vi "gui_control.vi"() -> ()   [LabVIEW 2020]
uses:
  <vilib>/Instr/_visa.llb/VISA Configure Serial Port (Instr).vi
panel:
  out "Connected":bool
  out "Response":string
  in  "CONNECTION":bool
  out "Bytes Read":u32
  in  "VISA Resource":refnum<visa-resource-name>="COM1"
  in  "Tab Control":enum32{"Page 1", "Page 2"}(tab)
  in  "End":timestamp caption="Day End" format="%<%H:%M>T"
  in  "Start":timestamp caption="Day Start" format="%<%H:%M>T"
  in  "SEND LED":bool caption="Boolean"
  out "Color Box":u32(colorbox)
  in  "R":u8
  in  "G":u8
  in  "B":u8
  in  "SEND RTC":bool caption="Boolean"
  in  "SEND INT":bool caption="Boolean"
  in  "INT 2":u8 caption="Brightness"
  out "Humidity":string caption="Humidity (%)"
  out "Temp":string caption="Temp (°C)"
  out "Temp 2":string caption="Temp (°C)"
  in  "B 2":u8 caption="B"
  in  "G 2":u8 caption="G"
  in  "R 2":u8 caption="R"
  out "Color Box 2":u32(colorbox)
  in  "SEND RTC 2":bool caption="Boolean"
  in  "SEND LED 2":bool caption="Boolean"
  in  "End 2":timestamp caption="Day End" format="%<%H:%M>T"
  in  "Start 2":timestamp caption="Day Start" format="%<%H:%M>T"
  in  "SEND INT 2":bool caption="Boolean"
  in  "INT":u8 caption="Brightness"
  out "Humidity 2":string caption="Humidity (%)"
  # "Serial Monitor"
  # "--- Box 1 ---"
  # "Auto LED Timer"
  # "Manual Color Control"
  # "Climate Readings"
  # "--- Box 2 ---"
  # "Auto LED Timer"
  # "Manual Color Control"
  # "Climate Readings"
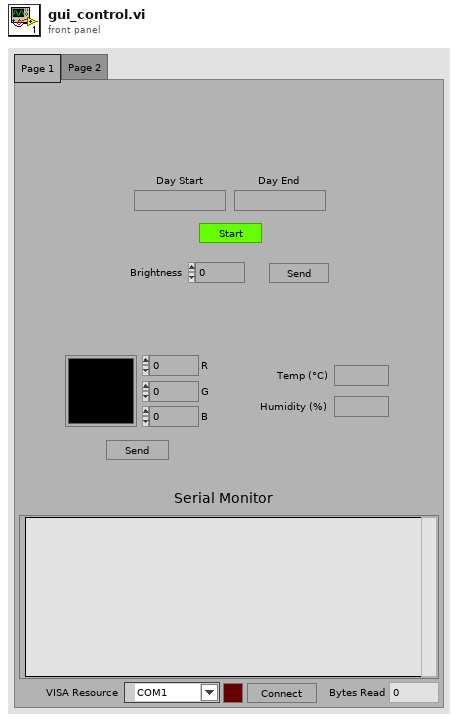
[diagram p1: front panel]
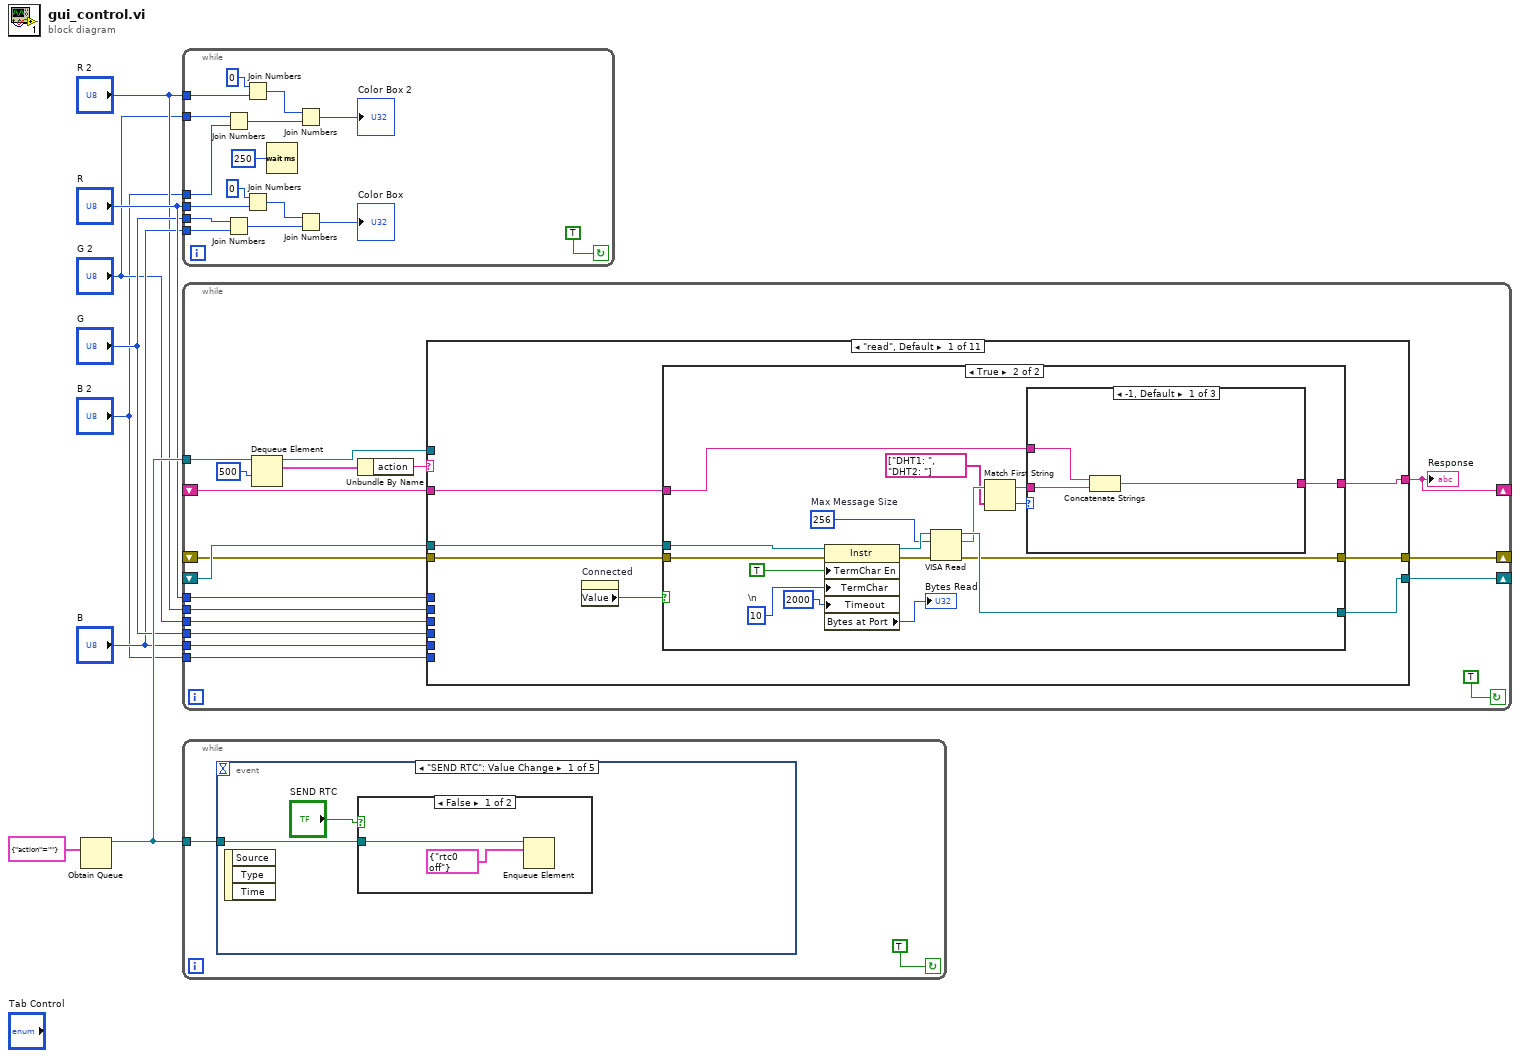
[diagram p0: block diagram]
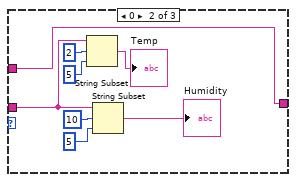
[diagram p3: hidden frame]
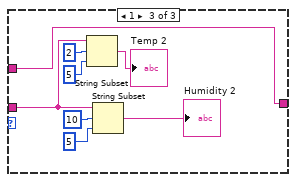
[diagram p4: hidden frame]
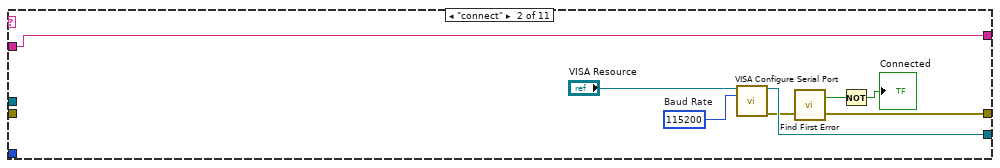
[diagram p5: hidden frame]
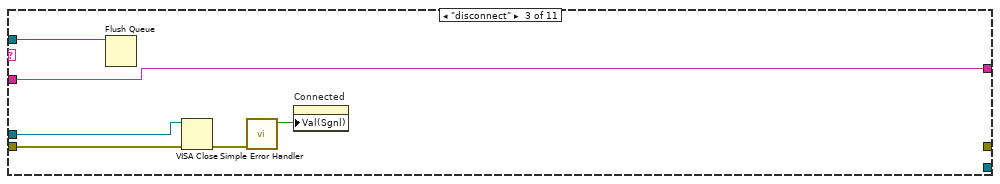
[diagram p6: hidden frame]
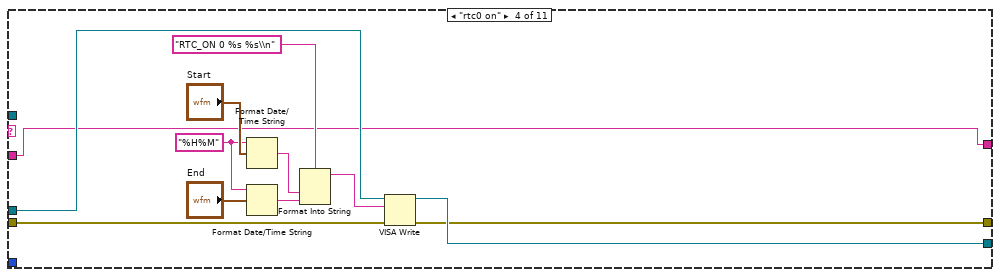
[diagram p7: hidden frame]
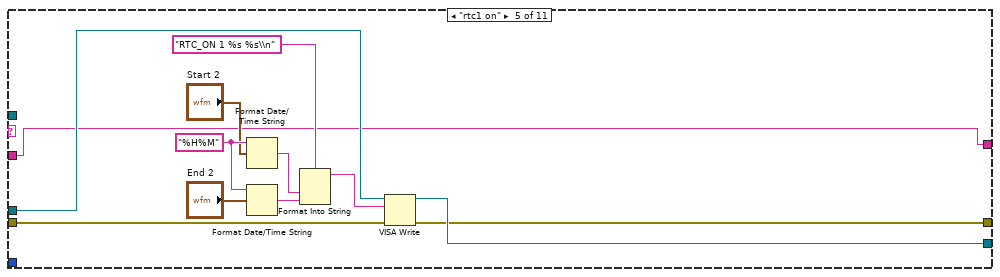
[diagram p8: hidden frame]
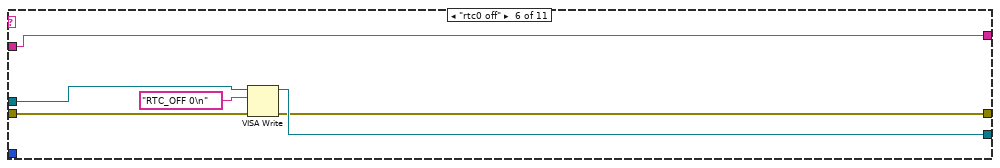
[diagram p9: hidden frame]
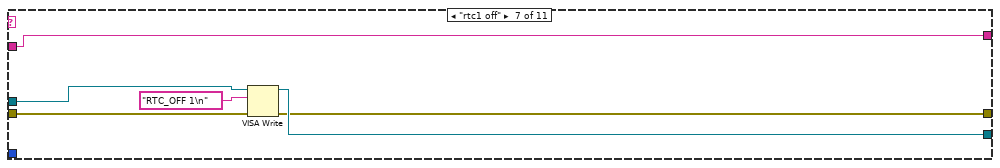
[diagram p10: hidden frame]
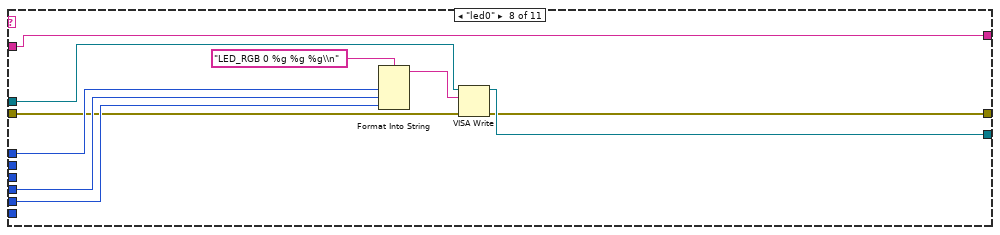
[diagram p11: hidden frame]
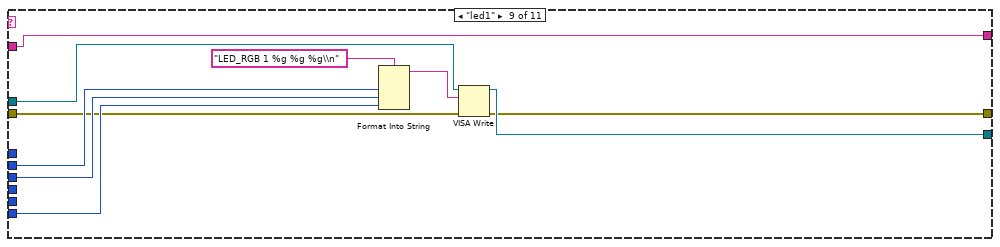
[diagram p12: hidden frame]
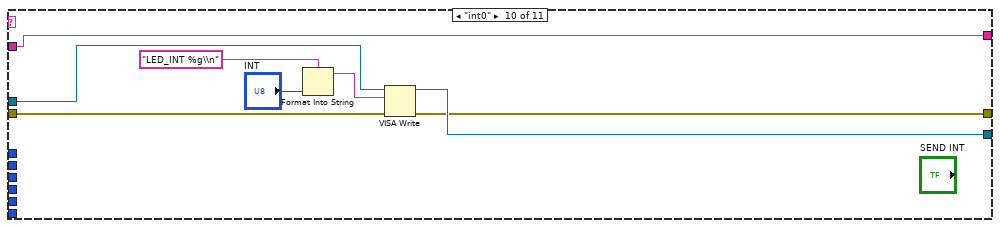
[diagram p13: hidden frame]
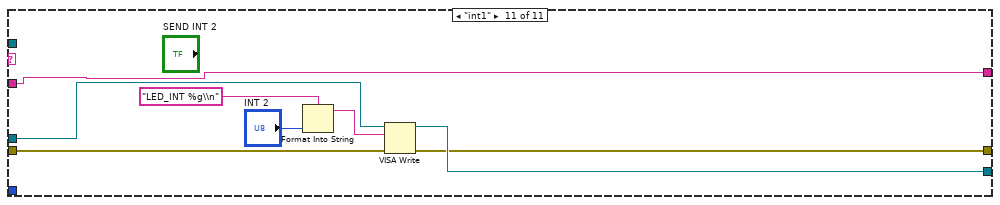
[diagram p14: hidden frame]
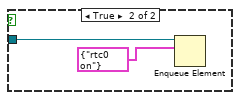
[diagram p15: hidden frame]
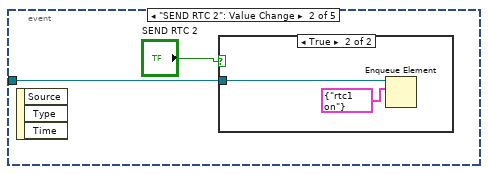
[diagram p16: hidden frame]
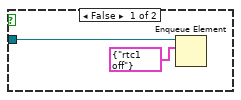
[diagram p17: hidden frame]
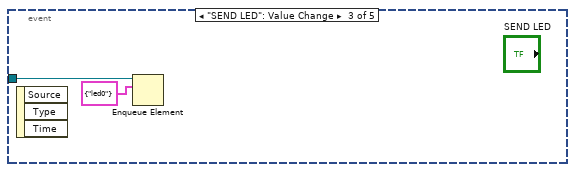
[diagram p18: hidden frame]
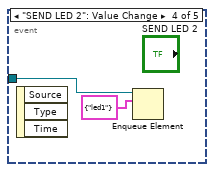
[diagram p19: hidden frame]
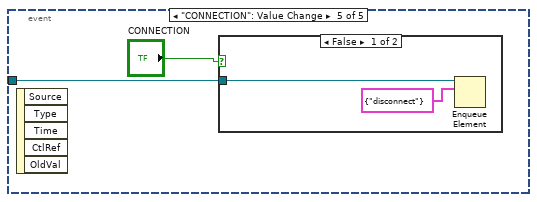
[diagram p20: hidden frame]
diagram:
  n1 = Obtain Queue(element data type=cluster{"action":string} {"action"=""}) -> (queue out=w7:refnum<queue>)  [unwired: 4 in, 2 out]
  n2 = while {
    tunnel: "R" -> [w18]
    tunnel: "G" -> [w17]
    tunnel: "B" -> [w16]
    tunnel: "R 2" -> [w14]
    tunnel: "G 2" -> [w12]
    tunnel: "B 2" -> [w11]
    stop <- TRUE continue-if-true
    n3 = Join Numbers(hi=w12, lo=w11) -> ((hi.lo)=w10:u16)
    n4 = Join Numbers(hi=w17, lo=w16) -> ((hi.lo)=w20:u16)
    n5 = Join Numbers(hi=u8 0, lo=w14) -> ((hi.lo)=w9:u16)
    n6 = Join Numbers(hi=u8 0, lo=w18) -> ((hi.lo)=w21:u16)
    n7 = Wait (ms)(milliseconds to wait=u32 250) -> ()  [unwired: 1 out]
    n8 = Join Numbers(hi=w9, lo=w10) -> ((hi.lo)=→"Color Box 2":u32)
    n9 = Join Numbers(hi=w21, lo=w20) -> ((hi.lo)=→"Color Box":u32)
  }
  n10 = while {
    tunnel: w7 -> [w42]
    shift-right: [w37] -> _
    shift-left: _ -> [w36]
    shift-right: [w35] -> _
    shift-left: _ -> [w34]
    tunnel: "R" -> [w33]
    tunnel: "G" -> [w32]
    tunnel: "B" -> [w31]
    tunnel: "R 2" -> [w30]
    tunnel: "G 2" -> [w29]
    tunnel: "B 2" -> [w28]
    shift-right: [w26] -> _
    shift-left: _ -> [w27]
    stop <- TRUE continue-if-true
    n11 = Dequeue Element(queue=w42, timeout in ms (-1)=500) -> (queue out=w38:refnum<queue>, element=w40:cluster{"action":string})  [unwired: 1 in, 2 out]
    n12 = Unbundle By Name(w40) -> ("action"=w39:string)
    n13 = case shown="\"read\", Default" w39 {
      tunnel: w38 -> [_ _ w97 _ _ _ _ _ _ _ _]
      tunnel: [w43 w92 _ w104 w117 w129 w135 w143 w153 w160 w169] -> w37
      tunnel: w36 -> [w49 _ w100 w105 w116 w130 w136 w144 w154 w161 w170]
      tunnel: [w47 w90 _ w102 w114 w127 w133 w138 w148 w158 w166] -> w35
      tunnel: w34 -> [w48 _ w98 w103 w115 w128 w134 w139 w149 w159 w167]
      tunnel: w33 -> [_ _ _ _ _ _ _ w142 _ _ _]
      tunnel: w32 -> [_ _ _ _ _ _ _ w141 _ _ _]
      tunnel: w31 -> [_ _ _ _ _ _ _ w140 _ _ _]
      tunnel: w30 -> [_ _ _ _ _ _ _ _ w152 _ _]
      tunnel: w29 -> [_ _ _ _ _ _ _ _ w151 _ _]
      tunnel: w28 -> [_ _ _ _ _ _ _ _ w150 _ _]
      tunnel: [w45 w87 w95 w101 w113 w126 w132 w137 w147 w157 w165] -> w26
      tunnel: w27 -> [w46 w87 w95 w101 w113 w126 w132 w137 w147 w157 w165]
      frame "read", Default {
        n14 = property on="Connected" class="Bool (strict)"() -> ("Value"=w44:bool)  [unwired: 2 in, 2 out]
        n15 = case shown="True" w44 {
          tunnel: w49 -> [_ w60]
          tunnel: w48 -> [w50 w59]
          tunnel: [w50 w57] -> w47
          tunnel: w46 -> [_ w52]
          tunnel: [_ w51] -> w45
          tunnel: [_ w58] -> w43
          frame False {
          }
          frame True {
            w64 = u32 256  # Max Message Size
            w62 = u8 10  # \n
            n16 = property class="Instr"(reference=w60, error in=w59, "TermChar En"=TRUE ("Message Based Settings:Termination Character Enable"), "TermChar"=w62, "Timeout"=u32 2000 ("General Settings:Timeout Value")) -> (reference out=w67:refnum<visa-resource-name>, error out=w66:errorcluster, "Bytes at Port"=→"Bytes Read":u32)
            n17 = VISA Read(VISA resource name=w67, byte count=w64, error in (no error)=w66) -> (VISA resource name out=w58:refnum<visa-resource-name>, read buffer=w56:string, error out=w57:errorcluster)  [unwired: 1 out]
            n18 = Match First String(2:string[] ["DHT1: ", "DHT2: "], 3:w56) -> (0:w55:i32, 1:w53:string)
            n19 = case shown="-1, Default" w55 {
              tunnel: w53 -> [w68 w72 w81]
              tunnel: w52 -> [w70 w78 w86]
              tunnel: [w69 w78 w86] -> w51
              frame -1, Default {
                n20 = Concatenate Strings(w70, w68) -> (w69:string)
              }
              frame 0 {
                n21 = String Subset(string=w72, offset (0)=2, length (rest)=5) -> (substring=→"Temp":string)
                n22 = String Subset(string=w72, offset (0)=10, length (rest)=5) -> (substring=→"Humidity":string)
              }
              frame 1 {
                n23 = String Subset(string=w81, offset (0)=2, length (rest)=5) -> (substring=→"Temp 2":string)
                n24 = String Subset(string=w81, offset (0)=10, length (rest)=5) -> (substring=→"Humidity 2":string)
              }
            }
          }
        }
      }
      frame "connect" {
        w93 = u32 115200  # Baud Rate
        n25 = call-poly "VISA Configure Serial Port"("VISA resource name"="VISA Resource", "baud rate (9600)"=w93) -> ("VISA resource name out"=w92:refnum<visa-resource-name>, "error out"=w91:errorcluster)  [unwired: 7 in, 5 out]
        n26 = call <vilib>:"Find First Error.vi"("error in (no error)"=w91) -> ("error out"=w90:errorcluster, "error?"=w89:bool)  [unwired: 3 in]
        n27 = Not(x=w89) -> (.not. x?=→"Connected":bool)
      }
      frame "disconnect" {
        n28 = Flush Queue(queue=w97) -> ()  [unwired: 1 in, 3 out]
        n29 = VISA Close(VISA resource name=w100, error in (no error)=w98) -> (error out=w99:errorcluster)
        n30 = call <vilib>:"Simple Error Handler.vi"("error in (no error)"=w99) -> ("error?"=w96:bool)  [unwired: 1 in, 7 out]
        n31 = property on="Connected" class="Bool (strict)"("Val(Sgnl)"=w96) -> ()  [unwired: 2 in, 2 out]
      }
      frame "rtc0 on" {
        w106 = "%H%M"
        n32 = Format Date/Time String(time format string (%c)=w106, seconds (now)="Start") -> (date/time string=w112:string)  [unwired: 1 in]
        n33 = Format Date/Time String(time format string (%c)=w106, seconds (now)="End") -> (date/time string=w111:string)  [unwired: 1 in]
        n34 = Format Into String(format string="RTC_ON 0 %s %s\\n", w112, w111) -> (resulting string=w108:string)  [unwired: 2 in, 1 out]
        n35 = VISA Write(VISA resource name=w105, write buffer=w108, error in (no error)=w103) -> (VISA resource name out=w104:refnum<visa-resource-name>, error out=w102:errorcluster)  [unwired: 1 out]
      }
      frame "rtc1 on" {
        w122 = "%H%M"
        n36 = Format Date/Time String(time format string (%c)=w122, seconds (now)="Start 2") -> (date/time string=w120:string)  [unwired: 1 in]
        n37 = Format Date/Time String(time format string (%c)=w122, seconds (now)="End 2") -> (date/time string=w121:string)  [unwired: 1 in]
        n38 = Format Into String(format string="RTC_ON 1 %s %s\\n", w120, w121) -> (resulting string=w123:string)  [unwired: 2 in, 1 out]
        n39 = VISA Write(VISA resource name=w116, write buffer=w123, error in (no error)=w115) -> (VISA resource name out=w117:refnum<visa-resource-name>, error out=w114:errorcluster)  [unwired: 1 out]
      }
      frame "rtc0 off" {
        n40 = VISA Write(VISA resource name=w130, write buffer="RTC_OFF 0\n" ("format string"), error in (no error)=w128) -> (VISA resource name out=w129:refnum<visa-resource-name>, error out=w127:errorcluster)  [unwired: 1 out]
      }
      frame "rtc1 off" {
        n41 = VISA Write(VISA resource name=w136, write buffer="RTC_OFF 1\n" ("format string"), error in (no error)=w134) -> (VISA resource name out=w135:refnum<visa-resource-name>, error out=w133:errorcluster)  [unwired: 1 out]
      }
      frame "led0" {
        n42 = Format Into String(format string="LED_RGB 0 %g %g %g\\n", w142, w141, w140) -> (resulting string=w145:string)  [unwired: 2 in, 1 out]
        n43 = VISA Write(VISA resource name=w144, write buffer=w145, error in (no error)=w139) -> (VISA resource name out=w143:refnum<visa-resource-name>, error out=w138:errorcluster)  [unwired: 1 out]
      }
      frame "led1" {
        n44 = Format Into String(format string="LED_RGB 1 %g %g %g\\n", w152, w151, w150) -> (resulting string=w155:string)  [unwired: 2 in, 1 out]
        n45 = VISA Write(VISA resource name=w154, write buffer=w155, error in (no error)=w149) -> (VISA resource name out=w153:refnum<visa-resource-name>, error out=w148:errorcluster)  [unwired: 1 out]
      }
      frame "int0" {
        n46 = Format Into String(format string="LED_INT %g\\n", "INT") -> (resulting string=w162:string)  [unwired: 2 in, 1 out]
        n47 = VISA Write(VISA resource name=w161, write buffer=w162, error in (no error)=w159) -> (VISA resource name out=w160:refnum<visa-resource-name>, error out=w158:errorcluster)  [unwired: 1 out]
      }
      frame "int1" {
        n48 = Format Into String(format string="LED_INT %g\\n", "INT 2") -> (resulting string=w171:string)  [unwired: 2 in, 1 out]
        n49 = VISA Write(VISA resource name=w170, write buffer=w171, error in (no error)=w167) -> (VISA resource name out=w169:refnum<visa-resource-name>, error out=w166:errorcluster)  [unwired: 1 out]
      }
    }
    "Response" <- w26
  }
  n50 = while {
    tunnel: w7 -> [w174]
    stop <- TRUE continue-if-true
    n51 = event shown="[0] \"SEND RTC\": Value Change" {
      selector: _ -> [_ _ _ _ _]
      dyn-events: _ -> [_ _ _ _ _]
      timeout: _ -> [_ _ _ _ _]
      tunnel: w174 -> [w175 w181 w187 w189 w192]
      event "SEND RTC": Value Change {
        n52 = event-data() -> ()  [unwired: 1 in, 3 out]
        n53 = case shown="False" "SEND RTC" {
          tunnel: w175 -> [w177 w179]
          frame False {
            n54 = Enqueue Element(queue=w177, element=cluster{"action":string} {"action"="rtc0 off"}) -> ()  [unwired: 2 in, 3 out]
          }
          frame True {
            n55 = Enqueue Element(queue=w179, element=cluster{"action":string} {"action"="rtc0 on"}) -> ()  [unwired: 2 in, 3 out]
          }
        }
      }
      event "SEND RTC 2": Value Change {
        n56 = event-data() -> ()  [unwired: 1 in, 3 out]
        n57 = case shown="True" "SEND RTC 2" {
          tunnel: w181 -> [w183 w185]
          frame False {
            n58 = Enqueue Element(queue=w183, element=cluster{"action":string} {"action"="rtc1 off"}) -> ()  [unwired: 2 in, 3 out]
          }
          frame True {
            n59 = Enqueue Element(queue=w185, element=cluster{"action":string} {"action"="rtc1 on"}) -> ()  [unwired: 2 in, 3 out]
          }
        }
      }
      event "SEND LED": Value Change {
        n60 = event-data() -> ()  [unwired: 1 in, 3 out]
        n61 = Enqueue Element(queue=w187, element=cluster{"action":string} {"action"="led0"}) -> ()  [unwired: 2 in, 3 out]
      }
      event "SEND LED 2": Value Change {
        n62 = event-data() -> ()  [unwired: 1 in, 3 out]
        n63 = Enqueue Element(queue=w189, element=cluster{"action":string} {"action"="led1"}) -> ()  [unwired: 2 in, 3 out]
      }
      event "CONNECTION": Value Change {
        n64 = event-data() -> ()  [unwired: 1 in, 5 out]
        n65 = case shown="False" "CONNECTION" {
          tunnel: w192 -> [w193 w196]
          frame False {
            n66 = Enqueue Element(queue=w193, element=cluster{"action":string} {"action"="disconnect"}) -> ()  [unwired: 2 in, 3 out]
          }
          frame True {
            n67 = Enqueue Element(queue=w196, element=cluster{"action":string} {"action"="connect"}) -> ()  [unwired: 2 in, 3 out]
          }
        }
      }
    }
  }
